vi "events2caseCamera.vi"(2 "Camara Controls Old":T3 {"Camera Parameters"."Pixel Format" items=["PIXEL_FORMAT_MONO8", "PIXEL_FORMAT_MONO16", "PIXEL_FORMAT_YUV422", "PIXEL_FORMAT_BAYER8_GRBG", "PIXEL_FORMAT_BAYER16_GRBG", "PIXEL_FORMAT_RGB24", "PIXEL_FORMAT_RGB48", "PIXEL_FORMAT_BAYER8_RGGB", "PIXEL_FORMAT_BAYER8_GBRG ", "PIXEL_FORMAT_BAYER8_BGGR ", "PIXEL_FORMAT_BAYER16_RGGB ", "PIXEL_FORMAT_BAYER16_GBRG", "PIXEL_FORMAT_BAYER16_BGGR", "PIXEL_FORMAT_RGB32"]}, 3 "Camara Controls New":T3 {"Camera Parameters"."Pixel Format" items=["PIXEL_FORMAT_MONO8", "PIXEL_FORMAT_MONO16", "PIXEL_FORMAT_YUV422", "PIXEL_FORMAT_BAYER8_GRBG", "PIXEL_FORMAT_BAYER16_GRBG", "PIXEL_FORMAT_RGB24", "PIXEL_FORMAT_RGB48", "PIXEL_FORMAT_BAYER8_RGGB", "PIXEL_FORMAT_BAYER8_GBRG ", "PIXEL_FORMAT_BAYER8_BGGR ", "PIXEL_FORMAT_BAYER16_RGGB ", "PIXEL_FORMAT_BAYER16_GBRG", "PIXEL_FORMAT_BAYER16_BGGR", "PIXEL_FORMAT_RGB32"]}) -> (0 "Cameara Cambio Array":T1(array[ring]), 1 "Camara Cambio?":bool)   [LabVIEW 2010]
uses:
  <vilib>/addons/PixeLINK/Low Level Functions/CAMERA_FEATURES.llb/TDPU-CameraFeatures-PixelFormat.ctl
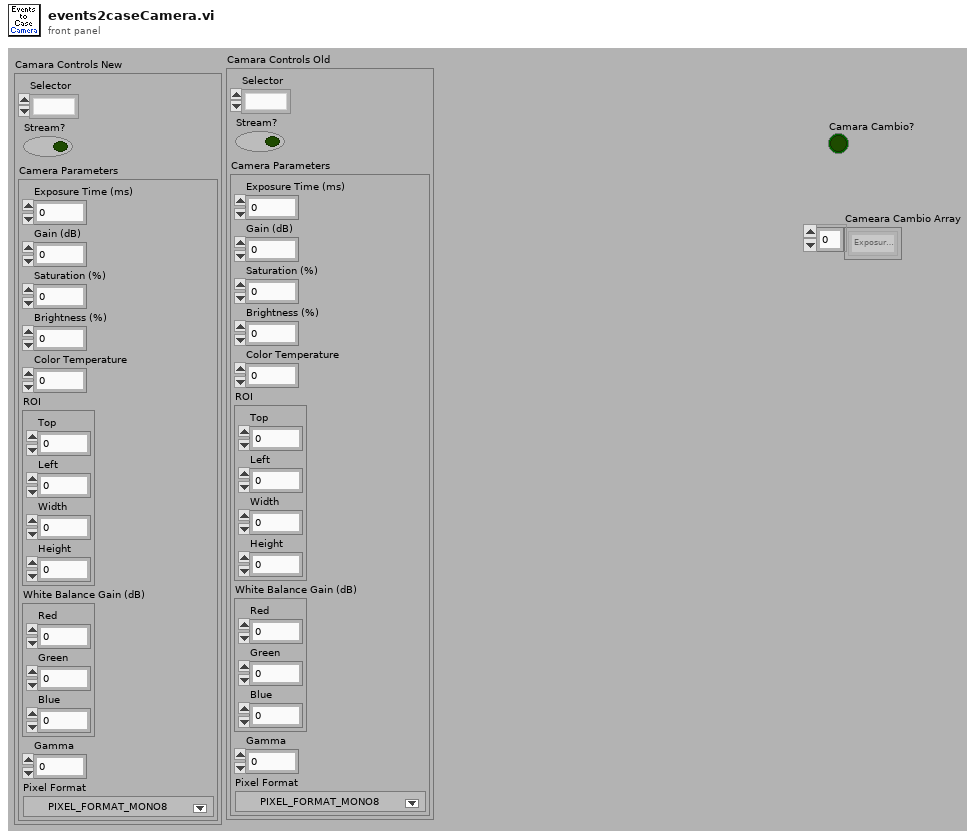
[diagram p1: front panel]
types:
  T1 = enum16{"Exposure Time (ms)", "Gain (dB)", "Saturation (%)", "Brightness (%)", "Color Temperature (%)", "ROI", "White Balance Gain (dB)", "Gamma", "Pixel Format", "Selector", "Stream", "Nothing"}[]
  T2 = typedef "TDPU-CameraFeatures-PixelFormat.ctl" = u16
  T3 = cluster{"Selector":u16, "Stream?":bool, "Camera Parameters":cluster{"Exposure Time (ms)":dbl, "Gain (dB)":dbl, "Saturation (%)":dbl, "Brightness (%)":dbl, "Color Temperature":dbl, "ROI":cluster{"Top":i32, "Left":i32, "Width":i32, "Height":i32}, "White Balance Gain (dB)":cluster{"Red":dbl, "Green":dbl, "Blue":dbl}, "Gamma":dbl, "Pixel Format":T2}}
  T4 = cluster{"Top":i32, "Left":i32, "Width":i32, "Height":i32}
  T5 = enum16{"Exposure Time (ms)", "Gain (dB)", "Saturation (%)", "Brightness (%)", "Color Temperature (%)", "ROI", "White Balance Gain (dB)", "Gamma", "Pixel Format", "Selector", "Stream", "Nothing"}
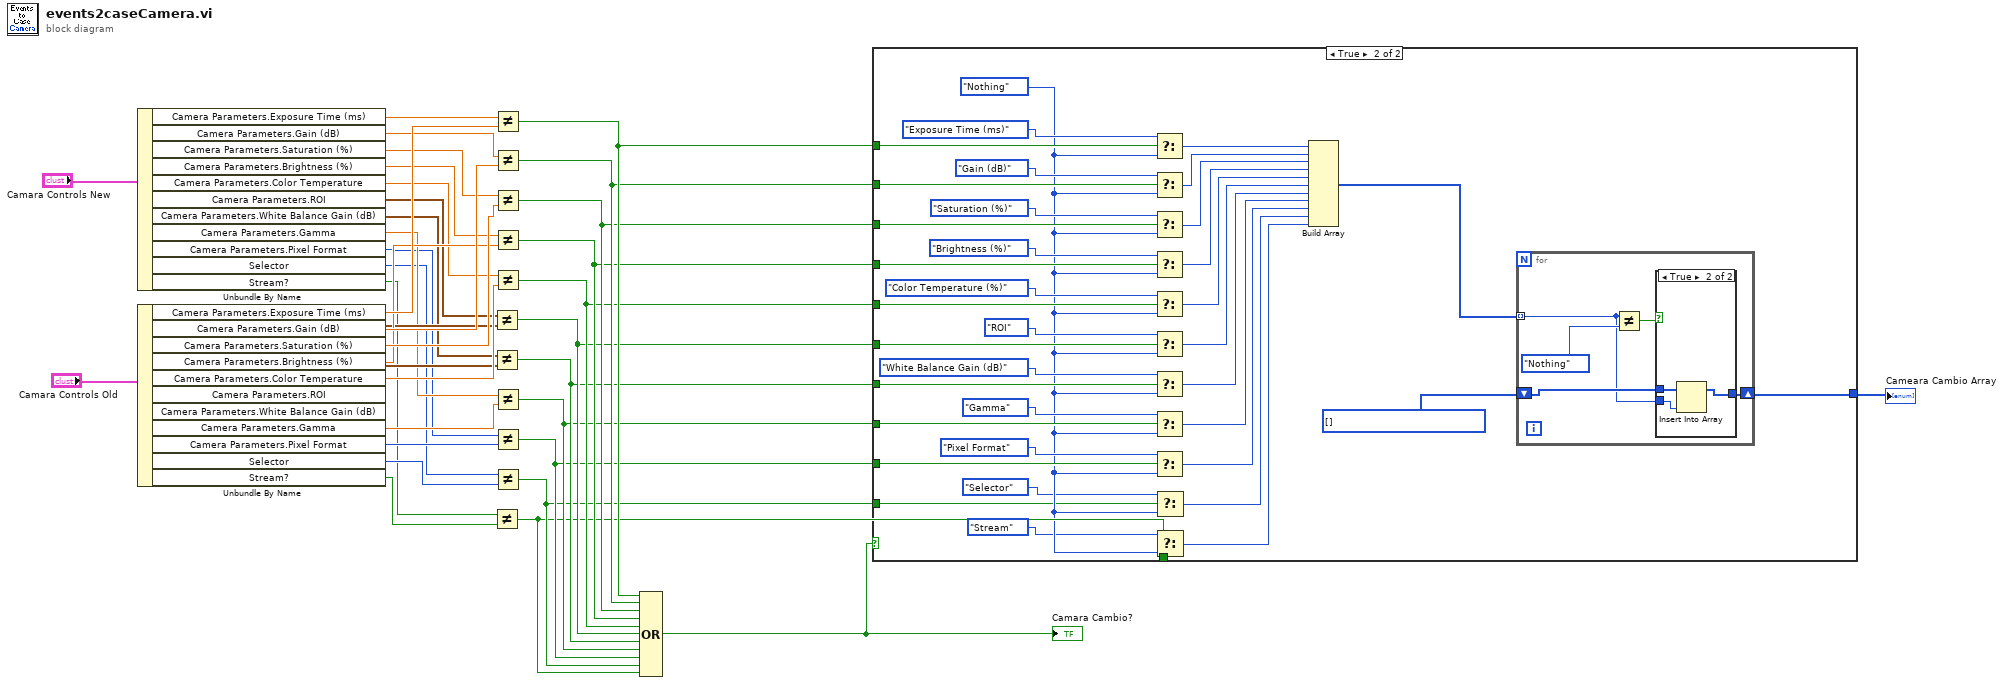
[diagram p0: block diagram]
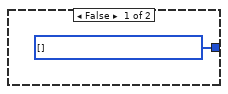
[diagram p2: hidden frame]
diagram:
  n1 = Unbundle By Name("Camara Controls New") -> ("Camera Parameters.Exposure Time (ms)"=w37:dbl, "Camera Parameters.Gain (dB)"=w35:dbl, "Camera Parameters.Saturation (%)"=w33:dbl, "Camera Parameters.Brightness (%)"=w31:dbl, "Camera Parameters.Color Temperature"=w29:dbl, "Camera Parameters.ROI"=w27:T4, "Camera Parameters.White Balance Gain (dB)"=w25:cluster{"Red":dbl, "Green":dbl, "Blue":dbl}, "Camera Parameters.Gamma"=w23:dbl, "Camera Parameters.Pixel Format"=w21:T2, "Selector"=w8:u16, "Stream?"=w6:bool)
  n2 = Unbundle By Name("Camara Controls Old") -> ("Camera Parameters.Exposure Time (ms)"=w36:dbl, "Camera Parameters.Gain (dB)"=w34:dbl, "Camera Parameters.Saturation (%)"=w32:dbl, "Camera Parameters.Brightness (%)"=w30:dbl, "Camera Parameters.Color Temperature"=w28:dbl, "Camera Parameters.ROI"=w26:T4, "Camera Parameters.White Balance Gain (dB)"=w24:cluster{"Red":dbl, "Green":dbl, "Blue":dbl}, "Camera Parameters.Gamma"=w22:dbl, "Camera Parameters.Pixel Format"=w20:T2, "Selector"=w7:u16, "Stream?"=w5:bool)
  n3 = Not Equal?(x=w27, y=w26) -> (x != y?=w14:bool)
  n4 = Not Equal?(x=w25, y=w24) -> (x != y?=w13:bool)
  n5 = Not Equal?(x=w6, y=w5) -> (x != y?=w3:bool)
  n6 = Not Equal?(x=w37, y=w36) -> (x != y?=w19:bool)
  n7 = Not Equal?(x=w35, y=w34) -> (x != y?=w18:bool)
  n8 = Not Equal?(x=w33, y=w32) -> (x != y?=w17:bool)
  n9 = Not Equal?(x=w31, y=w30) -> (x != y?=w16:bool)
  n10 = Not Equal?(x=w29, y=w28) -> (x != y?=w15:bool)
  n11 = Not Equal?(x=w23, y=w22) -> (x != y?=w12:bool)
  n12 = Not Equal?(x=w21, y=w20) -> (x != y?=w11:bool)
  n13 = Not Equal?(x=w8, y=w7) -> (x != y?=w4:bool)
  n14 = Compound Arithmetic op=OR(w19, w18, w17, w16, w15, w14, w13, w12, w11, w4, w3) -> (w2:bool)
  "Camara Cambio?" <- w2
  n15 = case shown="True" w2 {
    tunnel: w19 -> [_ w57]
    tunnel: w18 -> [_ w56]
    tunnel: w17 -> [_ w55]
    tunnel: w16 -> [_ w54]
    tunnel: w15 -> [_ w53]
    tunnel: w14 -> [_ w52]
    tunnel: w13 -> [_ w51]
    tunnel: w12 -> [_ w50]
    tunnel: w11 -> [_ w49]
    tunnel: w4 -> [_ w43]
    tunnel: w3 -> [_ w42]
    tunnel: [w38 w39] -> w1
    frame False {
      w38 = T1 [] items=["Exposure Time (ms)", "Gain (dB)", "Saturation (%)", "Brightness (%)", "Color Temperature (%)", "ROI", "White Balance Gain (dB)", "Gamma", "Pixel Format", "Selector", "Stream", "Nothing"]
    }
    frame True {
      w40 = T1 [] items=["Exposure Time (ms)", "Gain (dB)", "Saturation (%)", "Brightness (%)", "Color Temperature (%)", "ROI", "White Balance Gain (dB)", "Gamma", "Pixel Format", "Selector", "Stream", "Nothing"]
      w48 = T5."Nothing"
      n16 = Select(t=T5."Exposure Time (ms)", s=w57, f=w48) -> (s? t:f=w66:T5)
      n17 = Select(t=T5."Gain (dB)", s=w56, f=w48) -> (s? t:f=w65:T5)
      n18 = Select(t=T5."Saturation (%)", s=w55, f=w48) -> (s? t:f=w64:T5)
      n19 = Select(t=T5."Brightness (%)", s=w54, f=w48) -> (s? t:f=w63:T5)
      n20 = Select(t=T5."Color Temperature (%)", s=w53, f=w48) -> (s? t:f=w62:T5)
      n21 = Select(t=T5."ROI", s=w52, f=w48) -> (s? t:f=w61:T5)
      n22 = Select(t=T5."White Balance Gain (dB)", s=w51, f=w48) -> (s? t:f=w60:T5)
      n23 = Select(t=T5."Gamma", s=w50, f=w48) -> (s? t:f=w59:T5)
      n24 = Select(t=T5."Pixel Format", s=w49, f=w48) -> (s? t:f=w58:T5)
      n25 = Select(t=T5."Selector", s=w43, f=w48) -> (s? t:f=w45:T5)
      n26 = Select(t=T5."Stream", s=w42, f=w48) -> (s? t:f=w44:T5)
      n27 = Build Array(w66, w65, w64, w63, w62, w61, w60, w59, w58, w45, w44) -> (w41:T1)
      n28 = for {
        tunnel: w41 -> [w77] mode=indexing
        shift-right: [w76] -> w39
        shift-left: w40 -> [w78]
        n29 = Not Equal?(x=w77, y=T5."Nothing") -> (x != y?=w79:bool)
        n30 = case shown="True" w79 {
          tunnel: w78 -> [w81 w84]
          tunnel: w77 -> [_ w82]
          tunnel: [w81 w83] -> w76
          frame False {
          }
          frame True {
            n31 = Insert Into Array(array=w84, new element=w82) -> (w83:T1)  [unwired: 1 in]
          }
        }
      }
    }
  }
  "Cameara Cambio Array" <- w1
